vi "Get AI param from PGserver sh2.vi"(6 "conninfo":T2={"host"="localhost", "port"="5432", "client_encoding"="WIN1251", "dbname"="data", "user"="postgres", "password"=""}, 8 "error in (no error)":errorcluster, 9 "AIParamColumns":string[](array[string])=["instrument_gain", "instrument_offset", "time_const", "instrument_min_offset", "instrument_range_min", "process_range_min", "process_low_acd", "process_low_alr", "process_high_alr", "process_high_acd", "process_range_max", "instrument_range_max", "instrument_max_offset", "d", "input_register_min", "input_register_max", "input_pv_min", "input_pv_max", "fcode", "fcodef", "fcode_full", "fname", "process_units"], 10 "AIParamTable":string="fa_3", 11 "AIParameters":string[](array[string])) -> (0 "error out":errorcluster, 2 "Names table":string[][](array[string]), 3 "Parameters table":dbl[][](array[numeric]))   [LabVIEW 2019, in "Inputs.lvlib"]
uses:
  Inputs.lvlib
  Database/ctl/Coninfo.ctl
  Database/PostgreSQL2LabVIEW/libpqlv/src/PQfinish.vi
  Database/PostgreSQL2LabVIEW/libpqlv/src/PQconnectdb.vi
  Database/PostgreSQL2LabVIEW/libpqlv/src/PQerrorMessage.vi
  Database/PostgreSQL2LabVIEW/libpqlv/src/PQstatus.vi
  <vilib>/dlg_ctls.llb/Space Constant.vi
  Database/Progress.vi
  Database/PostgreSQL.lvlib
  Database/PostgreSQL2LabVIEW/libpqUtility64/libpqutility64.lvlib
  Database/PostgreSQL2LabVIEW/libpqUtility/libpqutility.lvlib
panel:
  out "PQStatus":T1(ring)
  # "fcode_full"
  # "fname"
  # "process_unit"
  # "time_const"
  # "instrument_min_offset"
  # "process_range_min"
  # "process_low_acd"
  # "instrument_range_max"
  # "d"
  # "input_register_min"
  # "input_register_max"
  # "input_pv_min"
  # "input_pv_max"
  # "fcodef"
  # "instrument_max_offset"
  # "instrument_range_min"
  # "process_range_max"
  # "instrument_offset"
  # "process_high_acd"
  # "process_high_alr"
  # "instrument_gain"
  # "process_low_alr"
  # "fcode"
  # "Names"
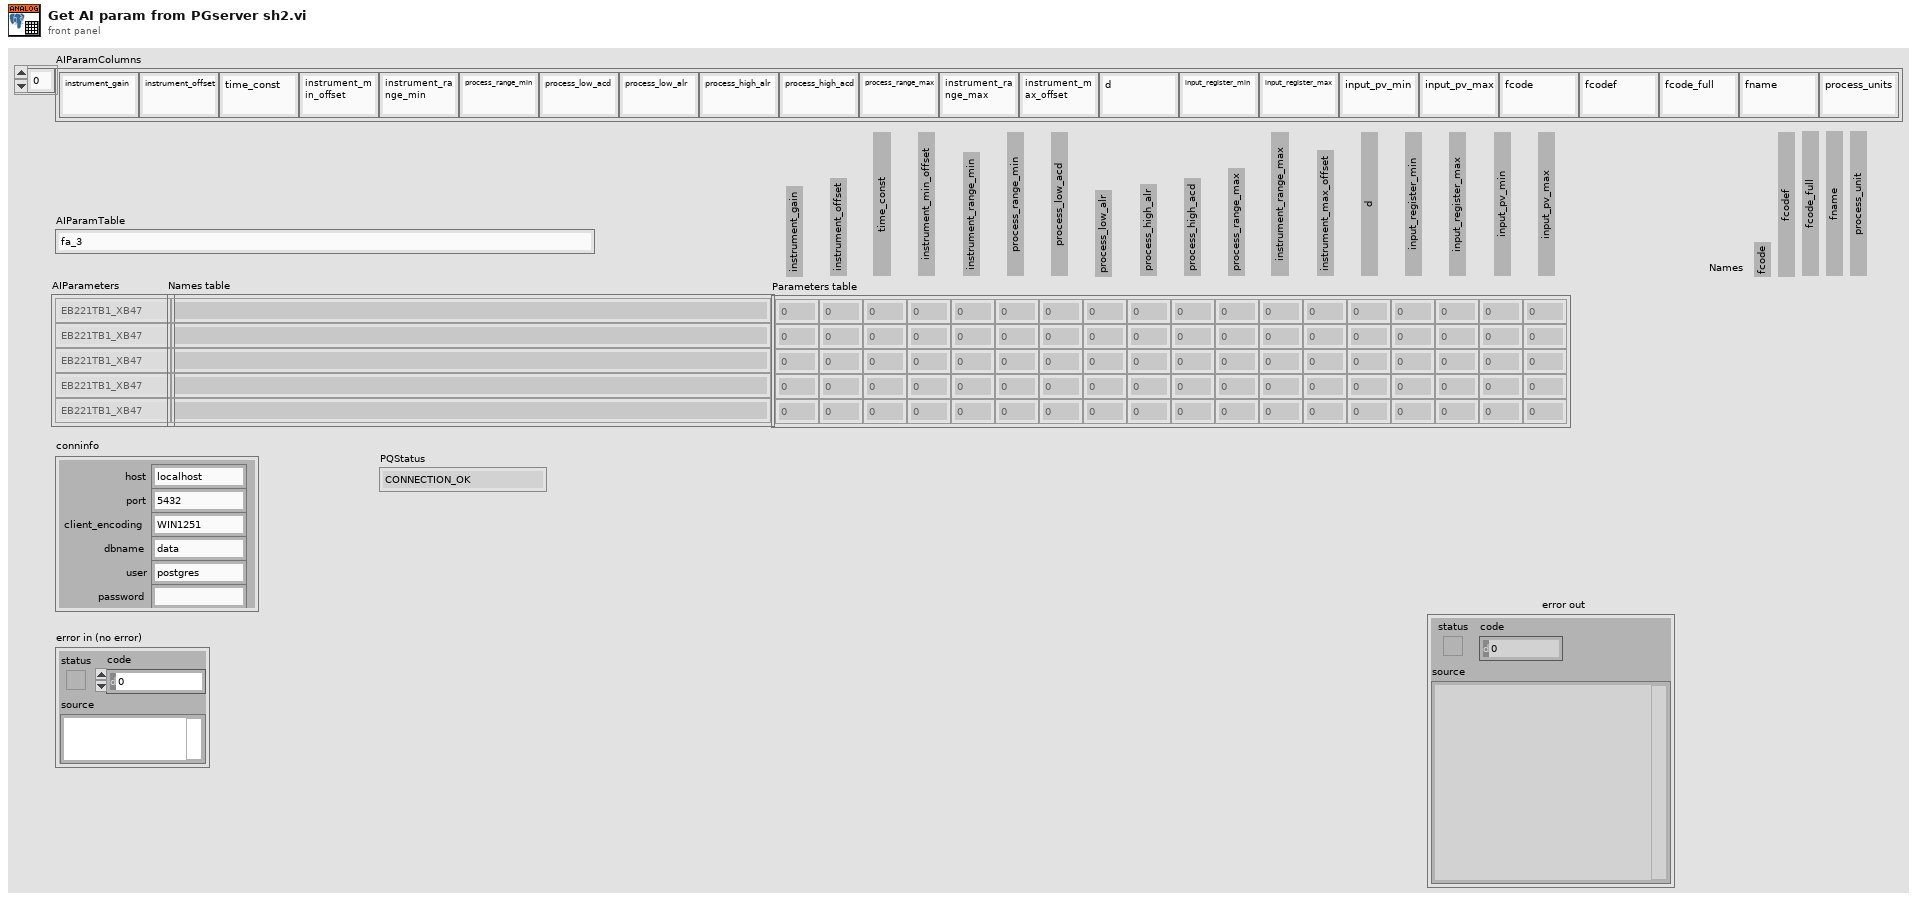
[diagram p1: front panel]
types:
  T1 = enum32{"CONNECTION_OK", "CONNECTION_BAD", "CONNECTION_STARTED", "CONNECTION_MADE", "CONNECTION_AWAITING_RESPONSE", "CONNECTION_AUTH_OK", "CONNECTION_SETENV", "CONNECTION_SSL_STARTUP", "CONNECTION_NEEDED"}
  T2 = typedef "PostgreSQL.lvlib/Coninfo.ctl" = cluster{"host":string, "port":string, "client_encoding":string, "dbname":string, "user":string, "password":string}
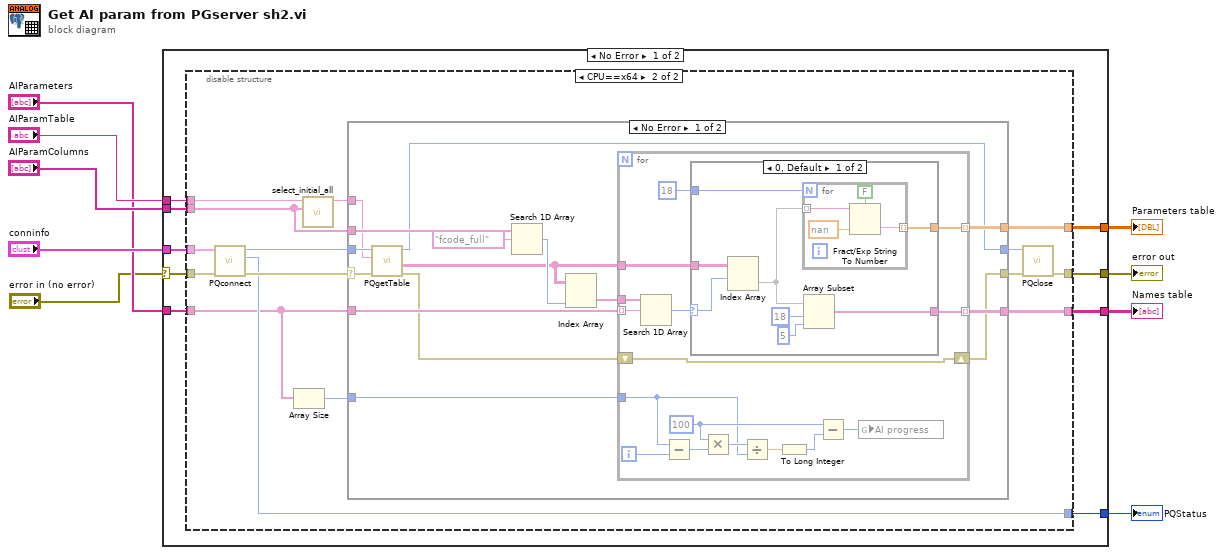
[diagram p0: block diagram]
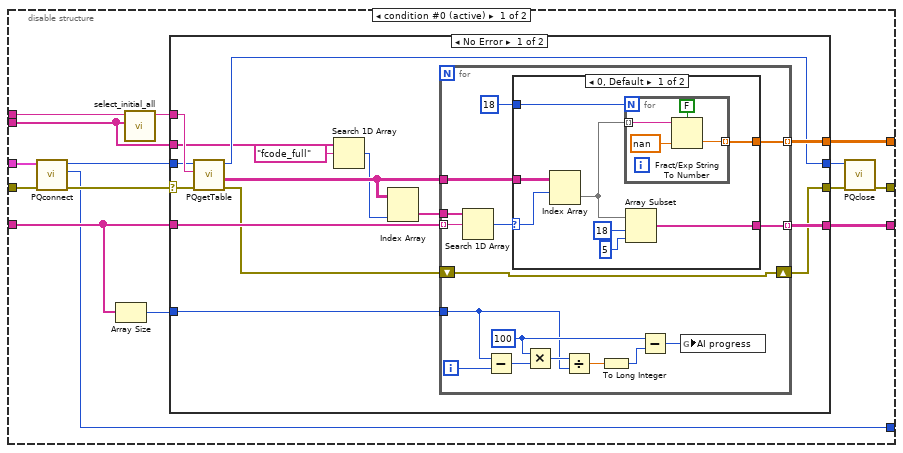
[diagram p2: hidden frame]
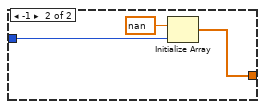
[diagram p3: hidden frame]
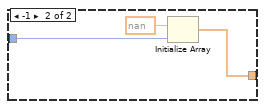
[diagram p5: hidden frame]
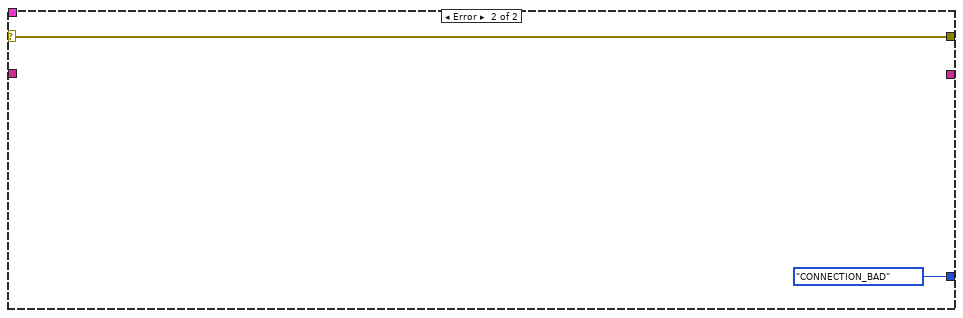
[diagram p7: hidden frame]
diagram:
  n1 = case shown="No Error" "error in (no error)" {
    selector: "error in (no error)" -> [w11 w146]
    tunnel: [w18 w146] -> w9
    tunnel: [w17 _] -> w8
    tunnel: [w16 _] -> w7
    tunnel: "AIParamColumns" -> [w15 _]
    tunnel: "conninfo" -> [w14 _]
    tunnel: "AIParamTable" -> [w13 _]
    tunnel: "AIParameters" -> [w12 _]
    tunnel: [w10 T1."CONNECTION_BAD" ("PQStatus")] -> w1
    frame No Error {
      n2 = disable-structure shown="CPU==x64" {
        disable-tunnel: [w20 w86] -> w18
        disable-tunnel: [w25 w85] -> w17
        disable-tunnel: [w24 w84] -> w16
        disable-tunnel: w15 -> [w19 w82]
        disable-tunnel: w14 -> [w29 w94]
        disable-tunnel: w13 -> [w27 w83]
        disable-tunnel: w12 -> [w26 w89]
        disable-tunnel: w11 -> [w28 w93]
        disable-tunnel: [w23 w90] -> w10
        frame condition #0 (active) {
          n3 = call "PQconnect.vi"("error in (no error)"=w28, "conninfo"=w29) -> ("error out"=w33:errorcluster, "PQStatus"=w23:T1, "conn"=w32:u32)  [unwired: 7 in]
          n4 = Array Size(array=w26) -> (size(s)=w31:i32)
          n5 = call "select_initial_all.vi"("Column table"=w19, "table"=w27) -> ("parameters"=w30:string)  [unwired: 8 in, 1 out]
          n6 = case shown="No Error" w33 {
            selector: w33 -> [w44 w81]
            tunnel: w26 -> [w45 _]
            tunnel: [w48 _] -> w25
            tunnel: [w47 _] -> w24
            tunnel: w31 -> [w46 _]
            tunnel: w32 -> [w42 w80]
            tunnel: w30 -> [w43 _]
            tunnel: [w34 w81] -> w21
            tunnel: [w41 w80] -> w22
            tunnel: w19 -> [w39 _]
            frame No Error {
              n7 = call "PQgetTable.vi"("error in"=w44, "query"=w43, "conn"=w42) -> ("error out"=w40:errorcluster, "Data"=w37:string[][], "conn_out"=w41:u32)  [unwired: 4 in, 2 out]
              n8 = Search 1D Array(1D array=w39, element="fcode_full" ("table")) -> (index of element=w36:i32)  [unwired: 1 in]
              n9 = Index Array(array=w37, index (col)=w36) -> (element=w35:string[])  [unwired: 1 in]
              n10 = for {
                tunnel: [w64] -> w47 mode=indexing
                tunnel: [w63] -> w48 mode=indexing
                tunnel: w46 -> [w55]
                tunnel: w45 -> [w52] mode=indexing
                shift-right: [w49] -> w34
                shift-left: w40 -> [w49]
                tunnel: w37 -> [w53]
                tunnel: w35 -> [w51]
                i -> [w56]
                w60 = 100 ("y")
                n11 = Search 1D Array(1D array=w51, element=w52) -> (index of element=w50:i32)  [unwired: 1 in]
                n12 = Subtract(x=w55, y=w56) -> (x-y=w59:i32)
                n13 = case shown="0, Default" w50 {
                  selector: w50 -> [w65 _]
                  tunnel: [w66 w78] -> w63
                  tunnel: 18 ("y") -> [w69 w77]
                  tunnel: w53 -> [w68 _]
                  tunnel: [w70 _] -> w64
                  frame 0, Default {
                    n14 = Index Array(array=w68, index (row)=w65) -> (element=w67:string[])  [unwired: 1 in]
                    n15 = for {
                      N: w69 -> [_]
                      tunnel: w67 -> [w75] mode=indexing
                      tunnel: [w74] -> w66 mode=indexing
                      n16 = Fract/Exp String To Number(use system decimal point (T)=FALSE, string=w75, default (0 dbl)=nan) -> (number=w74:dbl)  [unwired: 1 in, 1 out]
                    }
                    n17 = Array Subset(array=w67, index=18, length=5) -> (w70:string[])
                  }
                  frame -1 {
                    n18 = Initialize Array(nan, w77) -> (w78:dbl[])
                  }
                }
                n19 = Multiply(x=w60, y=w59) -> (x*y=w62:i32)
                n20 = Divide(x=w62, y=w55) -> (x/y=w58:dbl)
                n21 = To Long Integer(number=w58) -> (32bit integer=w57:i32)
                n22 = Subtract(x=w60, y=w57) -> (x-y=w61:i32)
                n23 = global write "Progress.vi" "AI progress"(w61) -> ()
              }
            }
            frame Error {
            }
          }
          n24 = call "PQclose.vi"("error in (no error)"=w21, "conn"=w22) -> ("error out"=w20:errorcluster)  [unwired: 9 in]
        }
        frame condition #1 {
          n25 = call "PQconnect.vi"("error in (no error)"=w93, "conninfo"=w94) -> ("error out"=w91:errorcluster, "PQStatus"=w90:T1, "conn"=w92:u64)  [unwired: 7 in]
          n26 = Array Size(array=w89) -> (size(s)=w96:i32)
          n27 = call "select_initial_all.vi"("Column table"=w82, "table"=w83) -> ("parameters"=w95:string)  [unwired: 8 in, 1 out]
          n28 = case shown="No Error" w91 {
            selector: w91 -> [w101 w144]
            tunnel: w89 -> [w108 _]
            tunnel: [w111 _] -> w85
            tunnel: [w110 _] -> w84
            tunnel: w96 -> [w109 _]
            tunnel: w92 -> [w102 w143]
            tunnel: w95 -> [w100 _]
            tunnel: [w103 w144] -> w87
            tunnel: [w99 w143] -> w88
            tunnel: w82 -> [w107 _]
            frame No Error {
              n29 = call "PQgetTable.vi"("error in"=w101, "query"=w100, "conn"=w102) -> ("error out"=w97:errorcluster, "Data"=w98:string[][], "conn_out"=w99:u64)  [unwired: 4 in, 2 out]
              n30 = Search 1D Array(1D array=w107, element="fcode_full" ("table")) -> (index of element=w105:i32)  [unwired: 1 in]
              n31 = Index Array(array=w98, index (col)=w105) -> (element=w104:string[])  [unwired: 1 in]
              n32 = for {
                tunnel: [w127] -> w110 mode=indexing
                tunnel: [w126] -> w111 mode=indexing
                tunnel: w109 -> [w118]
                tunnel: w108 -> [w115] mode=indexing
                shift-right: [w112] -> w103
                shift-left: w97 -> [w112]
                tunnel: w98 -> [w116]
                tunnel: w104 -> [w114]
                i -> [w119]
                w123 = 100 ("y")
                n33 = Search 1D Array(1D array=w114, element=w115) -> (index of element=w113:i32)  [unwired: 1 in]
                n34 = Subtract(x=w118, y=w119) -> (x-y=w122:i32)
                n35 = case shown="0, Default" w113 {
                  selector: w113 -> [w128 _]
                  tunnel: [w129 w141] -> w126
                  tunnel: 18 ("y") -> [w132 w140]
                  tunnel: w116 -> [w131 _]
                  tunnel: [w133 _] -> w127
                  frame 0, Default {
                    n36 = Index Array(array=w131, index (row)=w128) -> (element=w130:string[])  [unwired: 1 in]
                    n37 = for {
                      N: w132 -> [_]
                      tunnel: w130 -> [w138] mode=indexing
                      tunnel: [w137] -> w129 mode=indexing
                      n38 = Fract/Exp String To Number(use system decimal point (T)=FALSE, string=w138, default (0 dbl)=nan) -> (number=w137:dbl)  [unwired: 1 in, 1 out]
                    }
                    n39 = Array Subset(array=w130, index=18, length=5) -> (w133:string[])
                  }
                  frame -1 {
                    n40 = Initialize Array(nan, w140) -> (w141:dbl[])
                  }
                }
                n41 = Multiply(x=w123, y=w122) -> (x*y=w125:i32)
                n42 = Divide(x=w125, y=w118) -> (x/y=w121:dbl)
                n43 = To Long Integer(number=w121) -> (32bit integer=w120:i32)
                n44 = Subtract(x=w123, y=w120) -> (x-y=w124:i32)
                n45 = global write "Progress.vi" "AI progress"(w124) -> ()
              }
            }
            frame Error {
            }
          }
          n46 = call "PQclose.vi"("error in (no error)"=w87, "conn"=w88) -> ("error out"=w86:errorcluster)  [unwired: 9 in]
        }
      }
    }
    frame Error {
    }
  }
  "error out" <- w9
  "Parameters table" <- w8
  "Names table" <- w7
  "PQStatus" <- w1
